vi "Write ctl.vi"(8 "error in":errorcluster, 10 "ctl":cluster{"P":dbl, "I":dbl, "D":dbl}, 11 "Update TEC PID in":refnum<class "Update TEC PID.lvclass">) -> (0 "error out":errorcluster, 3 "Update TEC PID out":refnum<class "Update TEC PID.lvclass">)   [LabVIEW 2015, in "Generic TEC.lvlib" / "Update TEC PID.lvclass"]
uses:
  Update TEC PID.lvclass
  Update TEC PID.lvclass/Update TEC PID.ctl
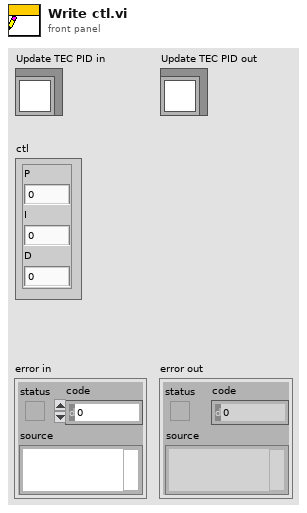
[diagram p1: front panel]
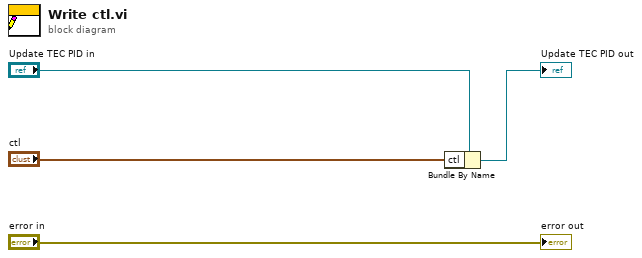
[diagram p0: block diagram]
diagram:
  n1 = Bundle By Name(cluster="Update TEC PID in", "ctl"="ctl") -> (→"Update TEC PID out":refnum<class "Update TEC PID.lvclass">)
  "error out" <- "error in"
